vi "1.vi"() -> ()   [LabVIEW 2017]
panel:
  out "Boolean 14":bool
  out "Boolean 13":bool
  out "Boolean 12":bool
  out "Boolean 11":bool
  out "Boolean 10":bool
  out "Boolean 9":bool
  out "Boolean 2":bool
  out "Boolean":bool
  in  "Boolean 8":bool
  in  "Boolean 1":bool
  in  "Boolean 7":bool
  in  "Boolean 6":bool
  in  "Boolean 5":bool
  in  "Boolean 4":bool
  in  "Boolean 3":bool
  in  "Boolean 2":bool
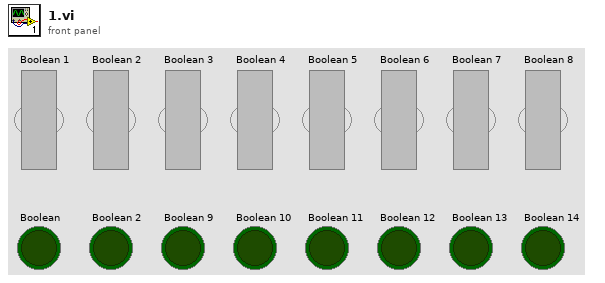
[diagram p1: front panel]
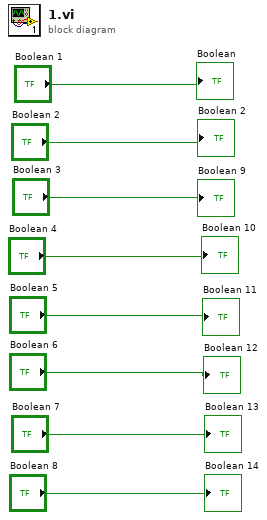
[diagram p0: block diagram]
diagram:
  "Boolean" <- "Boolean 1"
  "Boolean 2" <- "Boolean 2"
  "Boolean 9" <- "Boolean 3"
  "Boolean 10" <- "Boolean 4"
  "Boolean 11" <- "Boolean 5"
  "Boolean 12" <- "Boolean 6"
  "Boolean 13" <- "Boolean 7"
  "Boolean 14" <- "Boolean 8"
